vi "Write connect.vi"(8 "error in (no error)":errorcluster, 10 "connect":bool, 11 "Z_HSw in":refnum<class "Z_HSw.lvclass">) -> (0 "error out":errorcluster, 3 "Z_HSw out":refnum<class "Z_HSw.lvclass">)   [LabVIEW 2019, in "Z_HSw.lvclass"]
uses:
  Z_HSw.lvclass
  Z_HSw.lvclass/Z_HSw.ctl
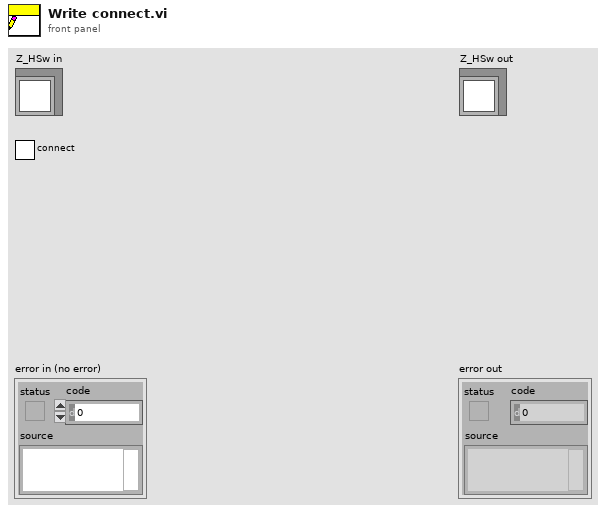
[diagram p1: front panel]
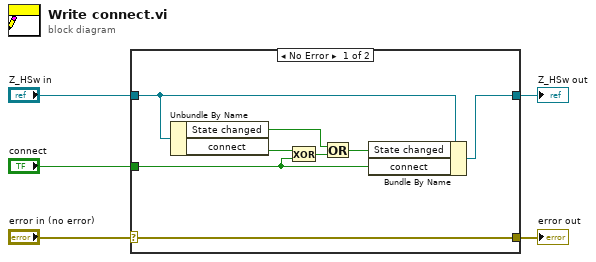
[diagram p0: block diagram]
diagram:
  n1 = case shown="No Error" "error in (no error)" {
    selector: "error in (no error)" -> [w13 w14]
    tunnel: [w13 w14] -> w4
    tunnel: [w12 w15] -> w2
    tunnel: "Z_HSw in" -> [w11 w15]
    tunnel: "connect" -> [w9 _]
    frame No Error {
      n2 = Unbundle By Name(w11) -> ("State changed"=w6:bool, "connect"=w10:bool)
      n3 = Exclusive Or(1:w9, 2:w10) -> (0:w8:bool)
      n4 = Or(x=w6, y=w8) -> (x .or. y?=w7:bool)
      n5 = Bundle By Name(cluster=w11, "State changed"=w7, "connect"=w9) -> (w12:refnum<class "Z_HSw.lvclass">)
    }
    frame Error {
    }
  }
  "error out" <- w4
  "Z_HSw out" <- w2
